vi "remove_ROI.vi"(8 "error in (no error)":errorcluster, 10 "RoiGeneric.lvclass":refnum<class "RoiGeneric.lvclass">, 11 "RoiCollection in":refnum<class "RoiCollection.lvclass">) -> (0 "error out":errorcluster, 3 "RoiCollection out":refnum<class "RoiCollection.lvclass">)   [LabVIEW 2010, in "RoiCollection.lvclass"]
uses:
  RoiCollection.lvclass
  RoiGeneric/RoiGeneric.lvclass
  RoiCollection.lvclass/RoiCollection.ctl
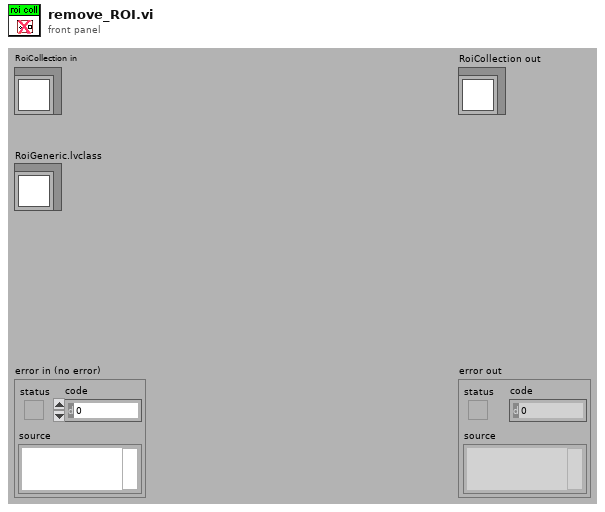
[diagram p1: front panel]
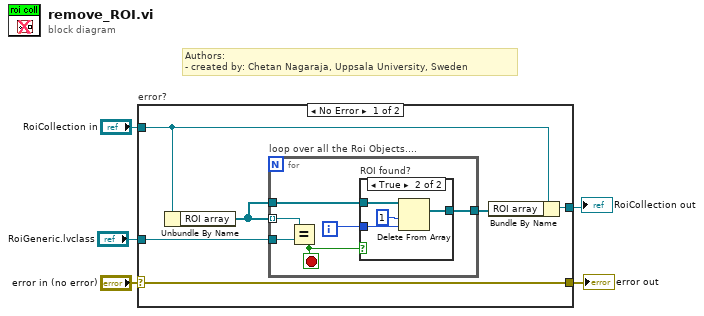
[diagram p0: block diagram]
diagram:
  # "Authors: \n- created by: Chetan Nagaraja, Uppsala University, Sweden"
  n1 = case "error?" shown="No Error" "error in (no error)" {
    selector: "error in (no error)" -> [w6 w24]
    tunnel: [w6 w24] -> w4
    tunnel: [w10 w23] -> w2
    tunnel: "RoiCollection in" -> [w11 w23]
    tunnel: "RoiGeneric.lvclass" -> [w9 _]
    frame No Error {
      n2 = Unbundle By Name(w11) -> ("ROI array"=w8:refnum<class "RoiGeneric.lvclass">[])
      n3 = for "loop over all the Roi Objects...." {
        tunnel: w8 -> [w16] mode=indexing
        tunnel: w9 -> [w17]
        tunnel: w8 -> [w15]
        tunnel: [w13] -> w7
        i -> [w14]
        stop <- w12 stop-if-true
        n4 = Equal?(x=w16, y=w17) -> (x = y?=w12:bool)
        n5 = case "ROI found?" shown="True" w12 {
          tunnel: w15 -> [w18 w22]
          tunnel: w14 -> [_ w21]
          tunnel: [w18 w19] -> w13
          frame False {
          }
          frame True {
            n6 = Delete From Array(array=w22, length=1, index=w21) -> (array with subset deleted=w19:refnum<class "RoiGeneric.lvclass">[])  [unwired: 1 out]
          }
        }
      }
      n7 = Bundle By Name(cluster=w11, "ROI array"=w7) -> (w10:refnum<class "RoiCollection.lvclass">)
    }
    frame Error {
    }
  }
  "error out" <- w4
  "RoiCollection out" <- w2
